vi "Create Downstream View SCM Spark Scene.vi"(2 "error in (no error)":errorcluster, 3 "Spark Coordinates (cm, rad, cm)":cluster{"r":sgl, "theta":sgl, "z":sgl}) -> (0 "error out":errorcluster, 1 "reference out":refnum<vi>)   [LabVIEW 2013, in "Breakdown Acoustics Controls.lvlib"]
uses:
  <vilib>/Utility/miscctls.llb/LV3DPointTypeDef.ctl
  <vilib>/picture/3D Picture Control/Object/Create Object (name).vi
  Breakdown Acoustics Controls.lvlib
  <vilib>/picture/3D Picture Control/NI_3D Picture Control.lvlib
panel:
  out "Cartesian\nCoordinates":cluster{"x":dbl, "y":dbl, "z":dbl}
  out "Spark Coordinates (cm, rad, rad)":cluster{"rho":dbl, "theta":dbl, "phi":dbl}
  out "Cavity Length (u)":sgl=1.2
  out "Cavity Radius (u)":sgl=1.2
  out "Graphical Units per Meter":dbl
  out "Cavity Downstream View":refnum<vi>(3d-picture)
  out "Spark Coordinates\n(cm, cm, cm)":T1
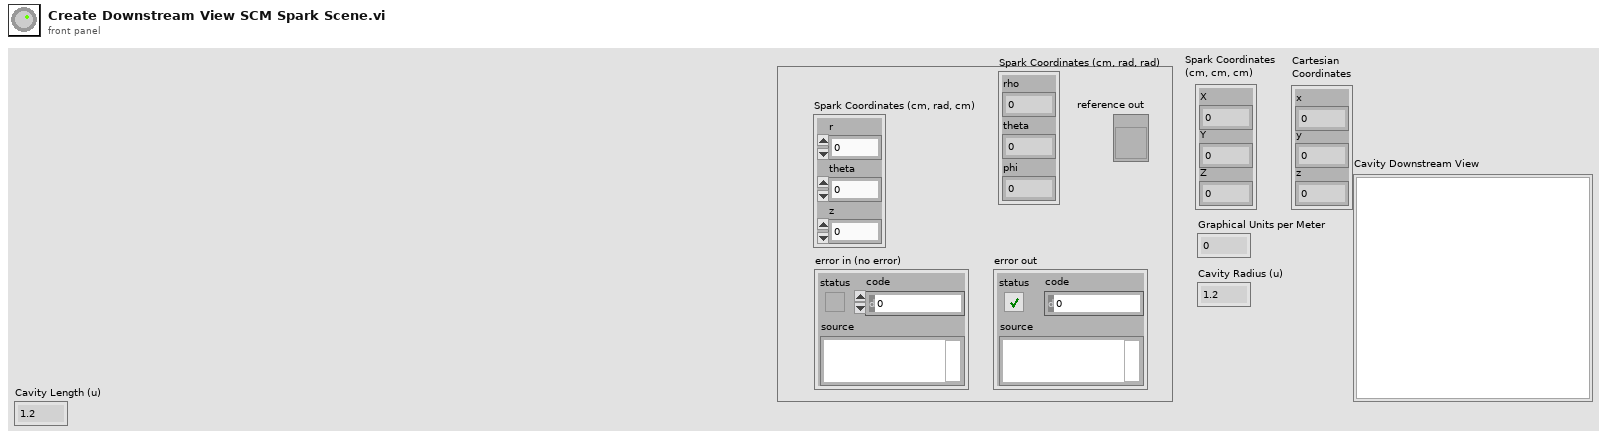
[diagram p1: front panel]
types:
  T1 = typedef "LV3DPointTypeDef.ctl" = cluster{"X":sgl, "Y":sgl, "Z":sgl}
  T2 = cluster{"Red":sgl, "Green":sgl, "Blue":sgl, "Alpha":sgl}
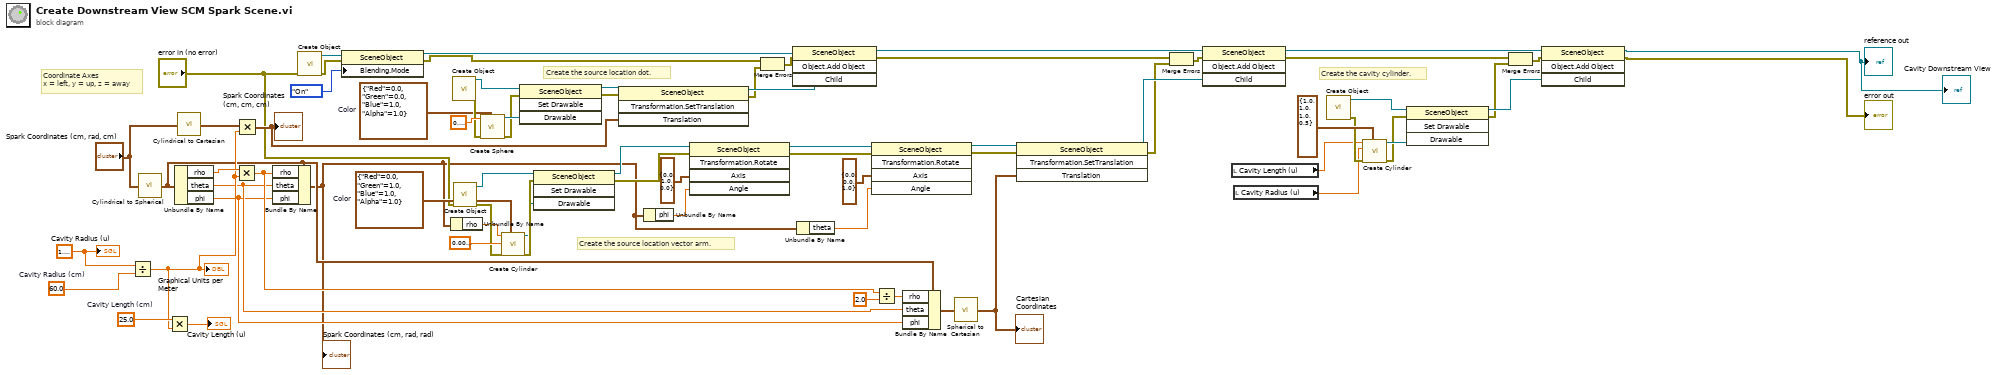
[diagram p0: block diagram]
diagram:
  w1 = T2 {"Red"=0.0, "Green"=0.0, "Blue"=1.0, "Alpha"=1.0}  # Color
  w18 = sgl 25.0  # Cavity Length (cm)
  w46 = T2 {"Red"=0.0, "Green"=1.0, "Blue"=1.0, "Alpha"=1.0}  # Color
  w58 = 60.0  # Cavity Radius (cm)
  w52 = sgl 1.2 ("Cavity Radius (u)")
  # "Coordinate Axes\nx = left, y = up, z = away"
  # "Create the source location vector arm."
  # "Create the source location dot."
  # "Create the cavity cylinder."
  n1 = Divide ("graphical units per meter")(x=w52, y=w58) -> (x/y=w17:dbl)
  "Graphical Units per Meter" <- w17
  n2 = call "Cylindrical to Spherical.vi"("Cylindrical\nCoordinates"="Spark Coordinates (cm, rad, cm)") -> ("Spherical\nCoordinates"=w7:cluster{"rho":dbl, "theta":dbl, "phi":dbl})  [unwired: 4 in]
  n3 = Multiply(x=w18, y=w17) -> (x*y=→"Cavity Length (u)":dbl)
  n4 = Unbundle By Name(w7) -> ("rho"=w22:dbl, "theta"=w9:dbl, "phi"=w8:dbl)
  n5 = call "Cylindrical to Cartesian.vi"("Cylindrical\nCoordinates"="Spark Coordinates (cm, rad, cm)") -> ("Cartesian\nCoordinates"=w20:cluster{"x":dbl, "y":dbl, "z":dbl})  [unwired: 4 in]
  n6 = Multiply(x=w22, y=w17) -> (x*y=w10:dbl)
  n7 = Multiply(x=w20, y=w17) -> (x*y=w19:cluster{"x":dbl, "y":dbl, "z":dbl})
  "Spark Coordinates\n(cm, cm, cm)" <- w19
  n8 = Bundle By Name(cluster=w7, "rho"=w10, "theta"=w9, "phi"=w8) -> (w4:cluster{"rho":dbl, "theta":dbl, "phi":dbl})
  "Spark Coordinates (cm, rad, rad)" <- w4
  n9 = call-poly <vilib>:"Create Object.vi"("error in (no error)"="error in (no error)") -> ("error out"=w66:errorcluster, "Scene:New Object"=w67:refnum<vi>)  [unwired: 9 in]
  n10 = property class="SceneObject"(reference=w67, error in=w66, "Blending.Mode"=enum16{"Inherit Value", "Off", "On"}."On" ("Blending:Mode")) -> (reference out=w65:refnum<vi>, error out=w54:errorcluster)
  n11 = Unbundle By Name(w4) -> ("rho"=w21:dbl)
  n12 = call-poly <vilib>:"Create Object.vi"() -> ("error out"=w51:errorcluster, "Scene:New Object"=w63:refnum<vi>)  [unwired: 10 in]
  n13 = call-poly <vilib>:"Create Object.vi"("error in (no error)"="error in (no error)") -> ("error out"=w43:errorcluster, "Scene:New Object"=w45:refnum<vi>)  [unwired: 9 in]
  n14 = call <vilib>:"Create Sphere.vi"("Color"=w1, "error in (no error)"=w51, "Radius"=sgl 0.1) -> ("error out"=w50:errorcluster, "New Sphere Refnum"=w69:refnum<vi>)  [unwired: 7 in]
  n15 = call <vilib>:"Create Cylinder.vi"("Color"=w46, "error in (no error)"=w43, "Radius"=sgl 0.01, "Height"=w21) -> ("error out"=w42:errorcluster, "New Cylinder Refnum"=w34:refnum<vi>)  [unwired: 6 in]
  n16 = invoke class="SceneObject" method="Set Drawable"(reference=w63, error in=w50, "Drawable"=w69) -> (reference out=w61:refnum<vi>, error out=w60:errorcluster)  [unwired: 1 in, 2 out]
  n17 = invoke class="SceneObject" method="Set Drawable"(reference=w45, error in=w42, "Drawable"=w34) -> (reference out=w32:refnum<vi>, error out=w31:errorcluster)  [unwired: 1 in, 2 out]
  n18 = invoke class="SceneObject" method="Transformation.SetTranslation"(reference=w61, error in=w60, "Translation"=w19) -> (reference out=w57:refnum<vi>, error out=w55:errorcluster)  [unwired: 1 in, 2 out]
  n19 = Unbundle By Name(w4) -> ("phi"=w24:dbl)
  n20 = invoke class="SceneObject" method="Transformation.Rotate"(reference=w32, error in=w31, "Axis"=T1 {"X"=0.0, "Y"=1.0, "Z"=0.0}, "Angle"=w24) -> (reference out=w38:refnum<vi>, error out=w37:errorcluster)  [unwired: 1 in, 3 out]
  n21 = Merge Errors(w54, w55) -> (w56:errorcluster)
  n22 = invoke class="SceneObject" method="Object.Add Object"(reference=w65, error in=w56, "Child"=w57) -> (reference out=w29:refnum<vi>, error out=w28:errorcluster)  [unwired: 1 in, 2 out]
  n23 = Unbundle By Name(w4) -> ("theta"=w23:dbl)
  n24 = invoke class="SceneObject" method="Transformation.Rotate"(reference=w38, error in=w37, "Axis"=T1 {"X"=0.0, "Y"=0.0, "Z"=1.0}, "Angle"=w23) -> (reference out=w36:refnum<vi>, error out=w35:errorcluster)  [unwired: 1 in, 3 out]
  n25 = Divide(x=w10, y=2.0) -> (x/y=w12:dbl)
  n26 = Bundle By Name(cluster=w7, "rho"=w12, "theta"=w9, "phi"=w8) -> (w6:cluster{"rho":dbl, "theta":dbl, "phi":dbl})
  n27 = call "Spherical to Cartesian.vi"("Spherical\nCoordinates"=w6) -> ("Cartesian\nCoordinates"=w5:cluster{"x":dbl, "y":dbl, "z":dbl})  [unwired: 4 in]
  "Cartesian\nCoordinates" <- w5
  n28 = invoke class="SceneObject" method="Transformation.SetTranslation"(reference=w36, error in=w35, "Translation"=w5) -> (reference out=w33:refnum<vi>, error out=w30:errorcluster)  [unwired: 1 in, 2 out]
  n29 = Merge Errors(w28, w30) -> (w41:errorcluster)
  n30 = invoke class="SceneObject" method="Object.Add Object"(reference=w29, error in=w41, "Child"=w33) -> (reference out=w27:refnum<vi>, error out=w26:errorcluster)  [unwired: 1 in, 2 out]
  n31 = local read "Cavity Length (u)"() -> (w15:sgl)
  n32 = local read "Cavity Radius (u)"() -> (w14:sgl)
  n33 = call-poly <vilib>:"Create Object.vi"() -> ("error out"=w49:errorcluster, "Scene:New Object"=w62:refnum<vi>)  [unwired: 10 in]
  n34 = call <vilib>:"Create Cylinder.vi"("Color"=T2 {"Red"=1.0, "Green"=1.0, "Blue"=1.0, "Alpha"=0.5}, "error in (no error)"=w49, "Radius"=w14, "Height"=w15) -> ("error out"=w48:errorcluster, "New Cylinder Refnum"=w68:refnum<vi>)  [unwired: 6 in]
  n35 = invoke class="SceneObject" method="Set Drawable"(reference=w62, error in=w48, "Drawable"=w68) -> (reference out=w59:refnum<vi>, error out=w47:errorcluster)  [unwired: 1 in, 2 out]
  n36 = Merge Errors(w26, w47) -> (w53:errorcluster)
  n37 = invoke class="SceneObject" method="Object.Add Object"(reference=w27, error in=w53, "Child"=w59) -> (reference out=→"reference out" →"Cavity Downstream View":refnum<vi>, error out=→"error out":errorcluster)  [unwired: 1 in, 2 out]
  "Cavity Radius (u)" <- w52
